vi "Cam1备份.vi"(1 "error in (no error)":errorcluster) -> (0 "error out":errorcluster caption="error in (no error)")   [LabVIEW 2018]
uses:
  <vilib>/vision/Image Controls.llb/IMAQ Image.ctl
  InOut/Reslut.vi
  VsyCam.dll
panel:
  in  "停止":bool
  in  "数据输出":i32[](listbox)
  out "通信":bool
  out "远场图":T1(plugin-control)
  in  "触发方式":enum8{"软件触发", "上升沿触发", "下降沿触发"}(ring)
  in  "曝光设置 us":i32 min=-1 max=420
  out "近场图":T1(plugin-control)
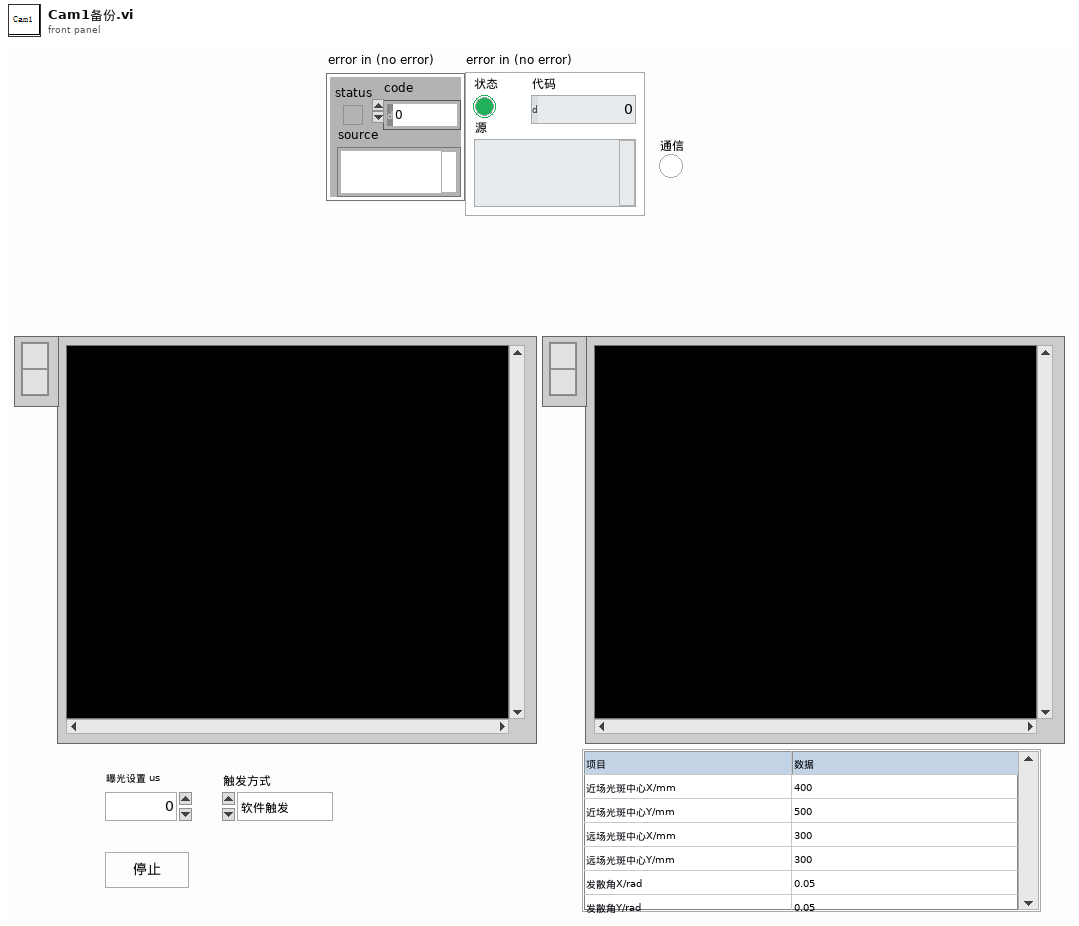
[diagram p1: front panel]
types:
  T1 = typedef "IMAQ Image.ctl" = refnum<image>
  T2 = enum16{"功率测量", "能量测量", "光谱测量", "时间波形", "偏振测量", "近远场"}
  T3 = cluster{"示波器":cluster{"Channel (0:Channel 1)":enum16{"Channel 1", "Channel 2", "Channel 3", "Channel 4"}, "电压范围":dbl, "触发电压":dbl, "时间范围":dbl, " 示波器VISA":refnum<visa-resource-name>}, "光谱仪":cluster{"Channel (0:Channel 1)":enum16{"Channel 1", "Channel 2", "Channel 3", "Channel 4"}, "电压范围":u64, "触发电压":u64, "时间范围":u64}, " 近场相机":cluster{"曝光时间":i32, "模拟增益":i32, "控制套接字":i32, "IP 地址":string, " 采集套接字":i32, "  版本号":i32, "ImageData":T1, "  增益最大":i32, "  增益最小":i32, " 曝光最大":i32, " 曝光最小":i32, " 帧速":i32, " 同步切换":i32, "  曝光缩放":i32}, " 偏振仪":cluster{"电压范围":u64, "触发电压":u64, "时间范围":u64, "波长范围":enum16{"可见光 400-700nm", "近红外 700-1100nm"}}, " 功率计":cluster{"通道":enum16{"Channel 1", "Channel 2"}, "工作波长":u32, "单位":u64, "时间范围":u64, "IP地址":string, "端口":u32}, "能量计":cluster{"通道":enum16{"Channel 1", "Channel 2"}, "工作波长":u32, "单位":u64, "时间范围":u64, "IP地址":string, "端口":u32, "能量计量程":enum16{"200uJ", "20uJ", "2uJ", "200nJ"}}, "电机":cluster{"Channel (0:Channel 1)":enum16{"Channel 1", "Channel 2", "Channel 3", "Channel 4"}, "电压范围":u64, "触发电压":u64, "时间范围":u64}, " 远场相机":cluster{"曝光时间":i32, "模拟增益":i32, "控制套接字":i32, "IP 地址":string, " 采集套接字":i32, "  版本号":i32, "ImageData":T1, "  增益最大":i32, "  增益最小":i32, " 曝光最大":i32, " 曝光最小":i32, " 帧速":i32, " 同步切换":i32, "  曝光缩放":i32}}
  T4 = cluster{"近场图":T1, " 远场图":T1, "发散角X/rad":dbl, "发散角Y/rad":dbl}
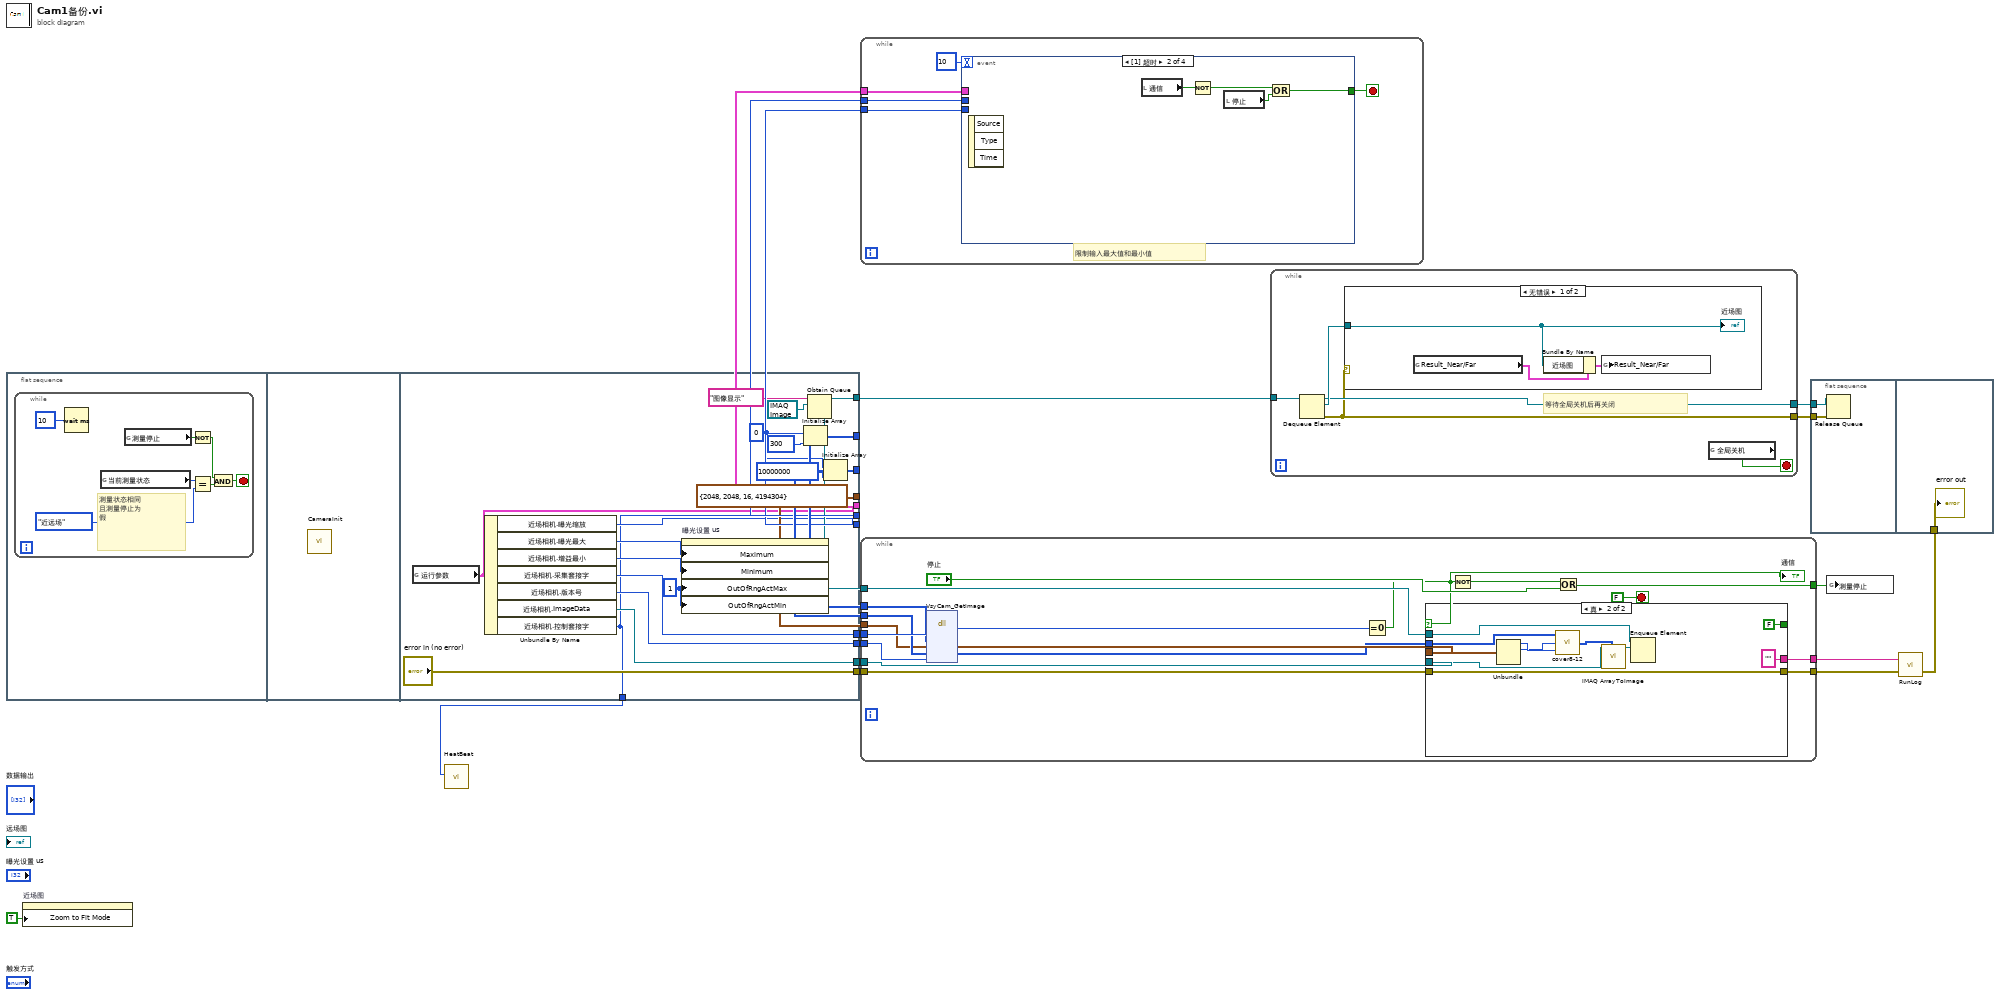
[diagram p0: block diagram]
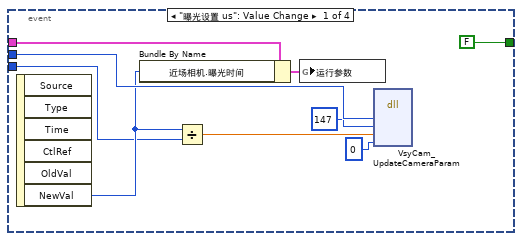
[diagram p3: hidden frame]
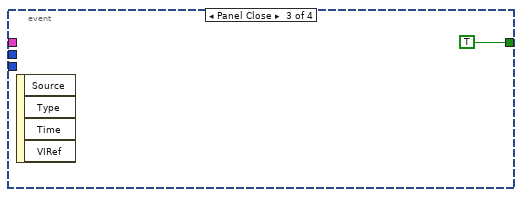
[diagram p4: hidden frame]
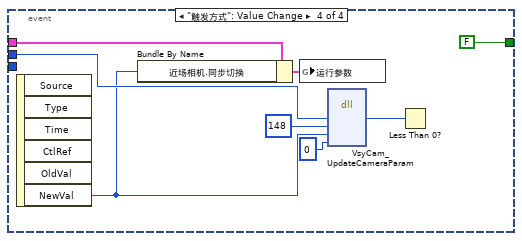
[diagram p5: hidden frame]
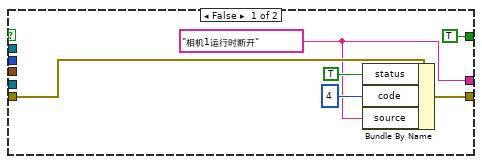
[diagram p6: hidden frame]
diagram:
  n1 = flat-sequence {
    tunnel: [w42] -> w19
    tunnel: [w41] -> w18
    tunnel: [w40] -> w17
    tunnel: [w39] -> w16
    tunnel: [w38] -> w15
    tunnel: [w27] -> w13
    tunnel: [w37] -> w12
    tunnel: ["error in (no error)"] -> w11
    tunnel: [w33] -> w8
    tunnel: [w32] -> w7
    tunnel: [cluster{i32, i32, i32, i32} {2048, 2048, 16, 4194304} ("簇")] -> w4
    tunnel: [w27] -> w1
    frame #0 {
      n2 = while {
        stop <- w23 stop-if-true
        # "测量状态相同\n且测量停止为\n假"
        n3 = Wait (ms)(milliseconds to wait=u32 10 ("等待时间（毫秒）")) -> ()  [unwired: 1 out]
        n4 = global read "参数.vi" "当前测量状态"() -> (w21:T2)
        n5 = global read "参数.vi" "测量停止"() -> (w24:bool)
        n6 = Not(x=w24) -> (.not. x?=w25:bool)
        n7 = Equal?(x=w21, y=T2."近远场" ("当前测量状态")) -> (x = y?=w20:bool)
        n8 = And(x=w25, y=w20) -> (x .and. y?=w23:bool)
      }
    }
    frame #1 {
      n9 = call "CameraInit.vi"() -> ()  [unwired: 1 in, 1 out]
    }
    frame #2 {
      w29 = u8 1 ("对超出界限的值的响应:最大值")
      w44 = u8 0
      n10 = global read "参数.vi" "运行参数"() -> (w32:T3)
      n11 = Unbundle By Name(w32) -> ("近场相机.曝光缩放"=w37:i32, "近场相机.曝光最大"=w31:i32, "近场相机.增益最小"=w30:i32, "近场相机.采集套接字"=w42:i32, "近场相机.版本号"=w41:i32, "近场相机.ImageData"=w38:T1, "近场相机.控制套接字"=w27:i32)
      n12 = property on="曝光设置 us" class="DigNum (严格)"("Maximum"=w31, "Minimum"=w30, "OutOfRngActMax"=w29, "OutOfRngActMin"=w29) -> ()  [unwired: 2 in, 2 out]
      n13 = Initialize Array(w44, 300) -> (w40:u8[])
      n14 = Obtain Queue(name (unnamed)="图像显示" ("名称（未命名）"), element data type=T1 refnum ("Image Out")) -> (queue out=w33:refnum<queue>)  [unwired: 3 in, 2 out]
      n15 = Initialize Array(w44, 10000000) -> (w39:u8[])
    }
  }
  n16 = property on="近场图" class="ImageControl"("Zoom to Fit Mode"=TRUE) -> ()  [unwired: 2 in, 2 out]
  n17 = call "HeatBeat.vi"("控制套接字"=w1) -> ()  [unwired: 11 in]
  n18 = while {
    tunnel: w7 -> [w50]
    tunnel: w13 -> [w49]
    tunnel: w12 -> [w48]
    stop <- w47 stop-if-true
    # "限制输入最大值和最小值"
    n19 = event shown="[1] 超时" {
      selector: _ -> [_ _ _ _]
      dyn-events: _ -> [_ _ _ _]
      timeout: 10 -> [_ _ _ _]
      tunnel: w50 -> [w59 _ _ w69]
      tunnel: w49 -> [w58 _ _ w72]
      tunnel: w48 -> [w54 _ _ _]
      tunnel: [FALSE w62 TRUE ("近场停止") FALSE] -> w47
      event "曝光设置 us": Value Change {
        n20 = event-data() -> ("NewVal"=w55:i32)  [unwired: 1 in, 5 out]
        n21 = Bundle By Name(cluster=w59, "近场相机.曝光时间"=w55) -> (w51:T3)
        n22 = Divide(x=w55, y=w54) -> (x/y=w53:dbl)
        n23 = global write "参数.vi" "运行参数"(w51) -> ()
        n24 = dll-call lib="PTH2?abs D做的项目航天测量软件相机\nVsyCam.dll" fn="VsyCam_UpdateCameraParam"("sockFd"=w58, "command"=147, "value"=w53, "ack"=0) -> ()  [unwired: 8 in, 2 out]
      }
      event Timeout {
        n25 = event-data() -> ()  [unwired: 1 in, 3 out]
        n26 = local read "通信"() -> (w61:bool)
        n27 = Not(x=w61) -> (.not. x?=w63:bool)
        n28 = local read "停止"() -> (w60:bool)
        n29 = Or(x=w63, y=w60) -> (x .or. y?=w62:bool)
      }
      event Panel Close {
        n30 = event-data() -> ()  [unwired: 1 in, 4 out]
      }
      event "触发方式": Value Change {
        n31 = event-data() -> ("NewVal"=w68:enum8{"软件触发", "上升沿触发", "下降沿触发"})  [unwired: 1 in, 5 out]
        n32 = Bundle By Name(cluster=w69, "近场相机.同步切换"=w68) -> (w65:T3)
        n33 = global write "参数.vi" "运行参数"(w65) -> ()
        n34 = dll-call lib="PTH2?abs D做的项目航天测量软件相机\nVsyCam.dll" fn="VsyCam_UpdateCameraParam"("sockFd"=w72, "command"=148, "value"=w68, "ack"=0) -> ("sockFd"=w67:i32)  [unwired: 7 in, 2 out]
        n35 = Less Than 0?(x=w67) -> ()  [unwired: 1 out]
      }
    }
  }
  n36 = while {
    tunnel: w19 -> [w90]
    tunnel: w18 -> [w89]
    tunnel: w17 -> [w88]
    tunnel: w16 -> [w86]
    tunnel: w15 -> [w82]
    tunnel: w4 -> [w85]
    tunnel: w11 -> [w81]
    tunnel: [w80] -> w10
    tunnel: [w79] -> w9
    tunnel: w8 -> [w78]
    tunnel: [w76] -> w3
    stop <- FALSE stop-if-true
    n37 = dll-call lib="PTH2?abs D做的项目航天测量软件相机\nVsyCam.dll" fn="VsyCam_GetImage" label="VsyCam_GetImageVsyCam_GetImage"("sockFd"=w90, "Header"=w88, "ImgInfo"=w85, "Data"=w86, "version"=w89) -> ("返回类型"=w87:i32, "ImgInfo"=w84:cluster{i32, i32, i32, i32}, "Data"=w83:u8[])  [unwired: 6 in, 2 out]
    n38 = Equal To 0?(x=w87) -> (x = 0?=w75:bool)
    "通信" <- w75
    n39 = case shown="真" w75 {
      tunnel: w84 -> [_ w107]
      tunnel: w83 -> [_ w106]
      tunnel: w82 -> [_ w103]
      tunnel: w81 -> [w96 w100]
      tunnel: [w93 w100] -> w80
      tunnel: [TRUE FALSE] -> _
      tunnel: [w91 "" ("source")] -> w79
      tunnel: w78 -> [_ w98]
      frame False {
        w91 = "相机1运行时断开" ("source")
        n40 = Bundle By Name(cluster=w96, "status"=TRUE, "code"=4, "source"=w91) -> (w93:errorcluster)
      }
      frame True {
        n41 = Unbundle(w107) -> (w105:i32, w104:i32)  [unwired: 2 out]
        n42 = call "cover8-12.vi"("H"=w105, "W"=w104, "Image Data"=w106) -> ("PIC Out"=w102:u16[][])
        n43 = call "IMAQ ArrayToImage"("Image Pixels (U16)"=w102, "Image"=w103) -> ("Image Out"=w97:T1)  [unwired: 8 in, 1 out]
        n44 = Enqueue Element(queue=w98, element=w97) -> ()  [unwired: 2 in, 3 out]
      }
    }
    n45 = Not(x=w75) -> (.not. x?=w74:bool)
    n46 = Or(x=w74, y="停止") -> (x .or. y?=w76:bool)
  }
  n47 = while {
    tunnel: w8 -> [w112]
    tunnel: [w110] -> w6
    tunnel: [w109] -> w2
    stop <- w108 stop-if-true
    # "等待全局关机后再关闭"
    n48 = Dequeue Element(queue=w112) -> (queue out=w110:refnum<queue>, element=w111:T1, error out=w109:errorcluster)  [unwired: 2 in, 1 out]
    n49 = case shown="无错误" w109 {
      tunnel: w111 -> [w114 _]
      frame No Error {
        n50 = global read "Reslut.vi" "Result_Near/Far"() -> (w115:T4)
        n51 = Bundle By Name(cluster=w115, "近场图"=w114) -> (w113:T4)
        n52 = global write "Reslut.vi" "Result_Near/Far"(w113) -> ()
        "近场图" <- w114
      }
      frame Error {
      }
    }
    n53 = global read "参数.vi" "全局关机"() -> (w108:bool)
  }
  n54 = flat-sequence {
    tunnel: w6 -> [w117]
    tunnel: w2 -> [w116]
    tunnel: w5 -> [w118]
    frame #0 {
      n55 = Release Queue(queue=w117, error in (no error)=w116) -> ()  [unwired: 1 in, 3 out]
    }
    frame #1 {
      "error out" <- w118
    }
  }
  n56 = global write "参数.vi" "测量停止"(w3) -> ()
  n57 = call "RunLog.vi"("error in"=w10, "Message"=w9) -> ("error out"=w5:errorcluster)  [unwired: 1 in]
